vi "Title_Data_save.vi"(6 "ErrorIndex":i32, 8 "Data in":T1, 11 "AllControls In":T2) -> (2 "数组":string[](array[string]))   [LabVIEW 2017]
uses:
  Ctrls/AllControls.ctl
  Ctrls/CSV_Data.ctl
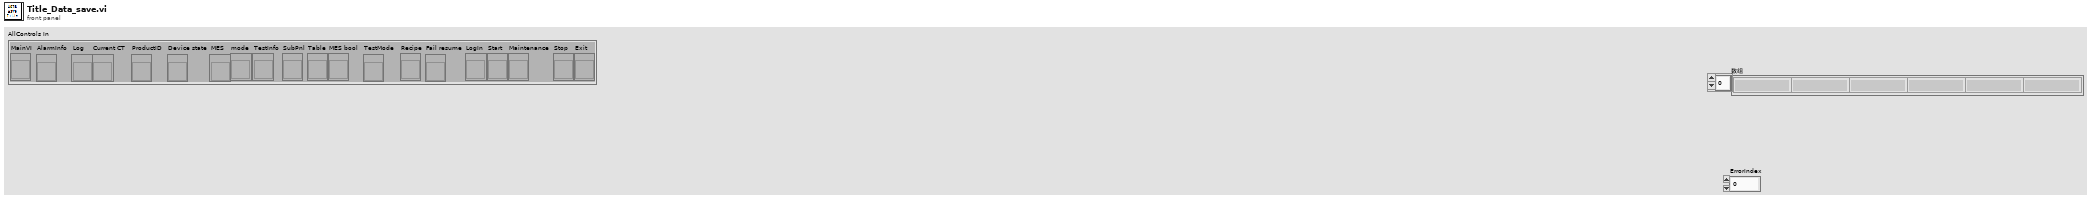
[diagram p1: front panel]
types:
  T1 = typedef "CSV_Data.ctl" = cluster{"SN":string, "Table":string[][], "Count":cluster{"Total":i32, "OK":i32, "NG":i32, "Yield":dbl}, "Start Time":timestamp, "daemon reference":refnum<k5>, "CT":dbl, "OK/NG":bool, "Station ID":string, "MES DDM SN":string, "MES PCBA SN":string, "Retest":string, "Attachment RFID detection":cluster{"UID":string, "tag content":string}, "SKU":string, "Plate_Diameter":string, "Alarm":string}
  T2 = typedef "AllControls.ctl" = cluster{"MainVI":refnum<vi>, "AlarmInfo":refnum<vi>, "Log":refnum<vi>, "Current CT":refnum<vi>, "ProductID":refnum<vi>, "Device state":refnum<vi>, "MES":refnum<vi>, "mode":refnum<vi>, "TestInfo":refnum<vi>, "SubPnl":refnum<vi>, "Table":refnum<vi>, "MES bool":refnum<vi>, "TestMode":refnum<vi>, "Recipe":refnum<vi>, "Fail resume":refnum<vi>, "LogIn":refnum<vi>, "Start":refnum<vi>, "Maintenance":refnum<vi>, "Stop":refnum<vi>, "Exit":refnum<vi>}
  T3 = typedef "HD Config.ctl" = cluster{" PC":cluster{"PC Address":u8[], "PC Port":i32}, "FCO":cluster{"COM":refnum<visa-resource-name>, "Baudrate":u32}, "DC Power ":cluster{"COM":refnum<visa-resource-name>, "Baudrate":u32}, "PW3336":cluster{"COM":refnum<visa-resource-name>, "Baudrate":u32}, "Lefoo":cluster{"COM":refnum<visa-resource-name>, "Baudrate":u32}, "AI Model":cluster{"COM":refnum<visa-resource-name>, "Baudrate":u32}, "DIPC":cluster{"COM":refnum<visa-resource-name>}, "RFID":cluster{"IP Address":string, "Port":u16, "Retry":u16}, "Motor":cluster{"COM":refnum<visa-resource-name>, "Baudrate":u32}, "Fail_resume_mode":bool, "GRR":bool}
  T4 = typedef "TesterInfo.ctl" = cluster{"Station Name":string, "Station Code":string, "ES NO.":string, "Tester ID":string, "PassMark Revision":string, "Rig ID":string, "Deamon_vision":string, "Project Name":string, "FFTesterPath":path, "Enable_User":bool, "Mode":enum16{"682"}, "MES":bool}
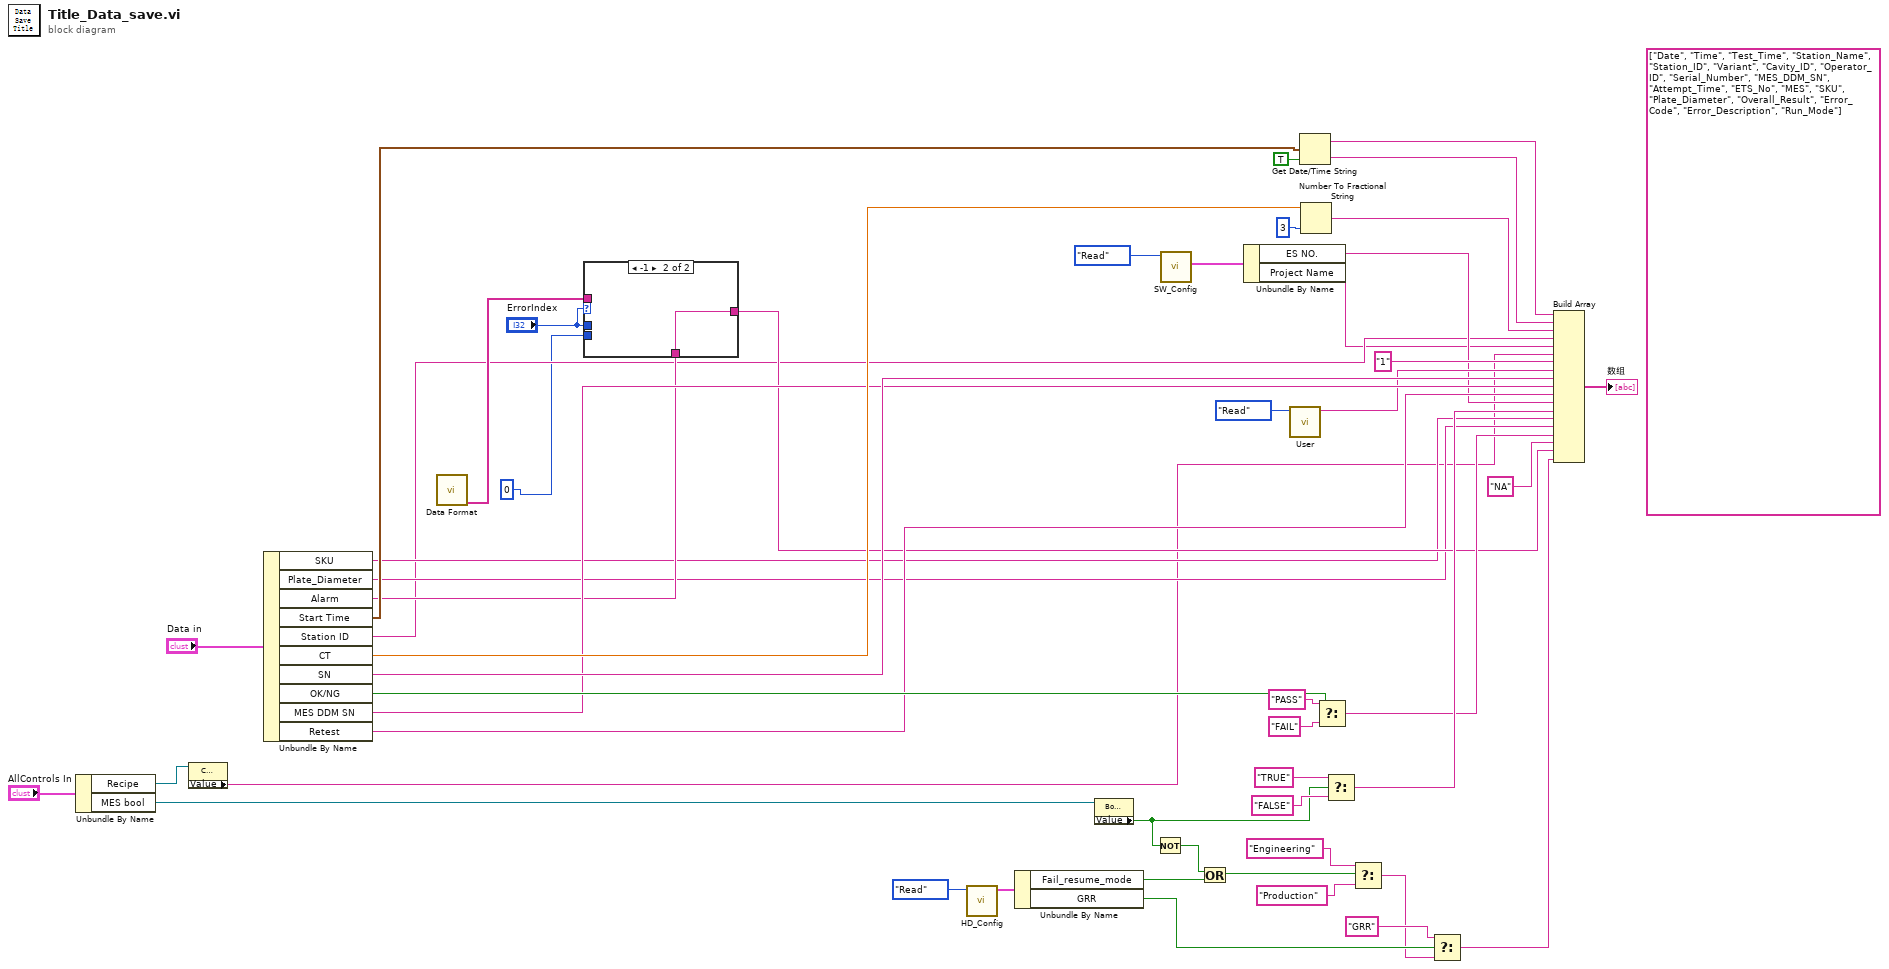
[diagram p0: block diagram]
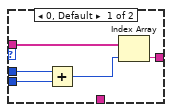
[diagram p2: hidden frame]
diagram:
  (unwired) string[] ["Date", "Time", "Test_Time", "Station_Name", "Station_ID", "Variant", "Cavity_ID", "Operator_ID", "Serial_Number", "MES_DDM_SN", "Attempt_Time", "ETS_No", "MES", "SKU", "Plate_Diameter", "Overall_Result", "Error_Code", "Error_Description", "Run_Mode"]
  n1 = Unbundle By Name("AllControls In") -> ("Recipe"=w13:refnum<vi>, "MES bool"=w36:refnum<vi>)
  n2 = property class="CmbBox"(reference=w13) -> ("Value"=w4:string)  [unwired: 1 in, 2 out]
  n3 = Unbundle By Name("Data in") -> ("SKU"=w6:string, "Plate_Diameter"=w5:string, "Alarm"=w7:string, "Start Time"=w10:timestamp, "Station ID"=w3:string, "CT"=w38:dbl, "SN"=w46:string, "OK/NG"=w34:bool, "MES DDM SN"=w24:string, "Retest"=w19:string)
  n4 = call "Data Format.vi"() -> ("title"=w12:string[])  [unwired: 10 in, 1 out]
  n5 = case shown="-1" "ErrorIndex" {
    tunnel: w12 -> [w56 _]
    tunnel: "ErrorIndex" -> [w55 _]
    tunnel: [w53 w57] -> w11
    tunnel: 0 -> [w52 _]
    tunnel: w7 -> [_ w57]
    frame 0, Default {
      n6 = Add(x=w55, y=w52) -> (x+y=w54:i32)
      n7 = Index Array(array=w56, index=w54) -> (element=w53:string)
    }
    frame -1 {
    }
  }
  n8 = call "HD_Config.vi"("Step"=enum16{"Initial", "Write", "Read"}."Read") -> ("HD Config out"=w32:T3)  [unwired: 9 in, 1 out]
  n9 = Unbundle By Name(w32) -> ("Fail_resume_mode"=w28:bool, "GRR"=w23:bool)
  n10 = property class="Bool (严格)"(reference=w36) -> ("Value"=w27:bool)  [unwired: 1 in, 2 out]
  n11 = Not(x=w27) -> (.not. x?=w25:bool)
  n12 = call "SW_Config.vi"("Step"=enum16{"Initial", "Write", "Read"}."Read") -> ("SW Config out"=w51:T4)  [unwired: 9 in, 1 out]
  n13 = Or(x=w25, y=w28) -> (x .or. y?=w26:bool)
  n14 = Unbundle By Name(w51) -> ("ES NO."=w16:string, "Project Name"=w2:string)
  n15 = call "User.vi"("Step"=enum16{"Initial", "Write", "Read"}."Read") -> ("User out"=w17:string)  [unwired: 9 in, 1 out]
  n16 = Get Date/Time String(seconds (now)=w10, want seconds? (F)=TRUE ("需要秒？(F)")) -> (date string=w40:string, time string=w41:string)  [unwired: 1 in]
  n17 = Number To Fractional String(number=w38, precision (6)=i16 3 ("精度(6)")) -> (F-format string=w43:string)  [unwired: 2 in]
  n18 = Select(t="PASS" ("真字符串"), s=w34, f="FAIL" ("假字符串")) -> (s? t:f=w14:string)
  n19 = Select(t="TRUE" ("真字符串"), s=w27, f="FALSE" ("假字符串")) -> (s? t:f=w15:string)
  n20 = Select(t="Engineering", s=w26, f="Production") -> (s? t:f=w21:string)
  n21 = Select(t="GRR", s=w23, f=w21) -> (s? t:f=w20:string)
  n22 = Build Array(w40, w41, w43, w3, w2, w4, "1" ("Cavity ID_L"), w17, w46, w24, w19, w16, w15, w6, w5, w14, "NA" ("element"), w11, w20) -> (→"数组":string[])
